vi "Union.vi"(8 "New headers":refnum<class "httpHeaders.lvclass">, 11 "Original headers":refnum<class "httpHeaders.lvclass">) -> (3 "Merged Headers":refnum<class "httpHeaders.lvclass">)   [LabVIEW 2020, in "httpClient.lvlib" / "httpHeaders.lvclass"]
uses:
  httpHeaders.lvclass
  httpHeaders.lvclass/httpHeaders.ctl
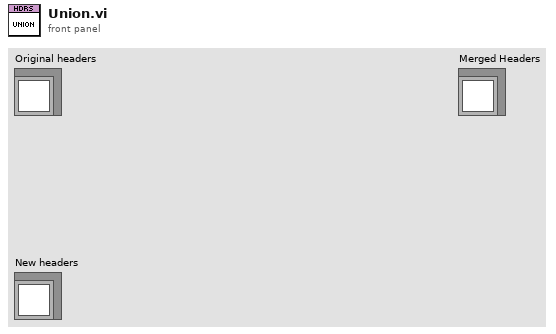
[diagram p1: front panel]
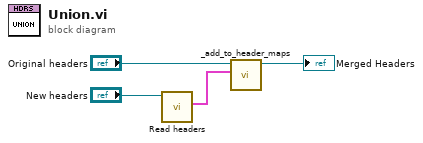
[diagram p0: block diagram]
diagram:
  n1 = call "Read headers.vi"("httpHeaders in"="New headers") -> ("headers"=w2:cluster{"header":string, "value":string}[])  [unwired: 8 in, 2 out]
  n2 = call "_add_to_header_maps.vi"("ordered headers"=w2, "httpHeaders in"="Original headers") -> ("httpHeaders out"=→"Merged Headers":refnum<class "httpHeaders.lvclass">)  [unwired: 9 in]
